vi "DataSocketOutput-Start.vi"(3 "error in (no error)":errorcluster, 4 "OutputRequest\nuser event refnum":T1, 5 "Configuration":T2) -> (0 "error out":errorcluster)   [LabVIEW 2015]
doc: "Starts the DataSocketOutput daemon running.\n\nIf the DataSocket URL is empty, then this will warn the user and then exit."
uses:
  DataSocketOutput-Configuration.ctl
  Typedefs/OutputRequest refnum.ctl
  Typedefs/OutputRequest.ctl
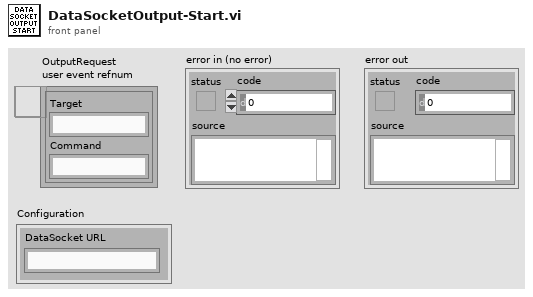
[diagram p1: front panel]
types:
  T1 = typedef "OutputRequest refnum.ctl" = refnum<user-event>
  T2 = typedef "DataSocketOutput-Configuration.ctl" = cluster{"DataSocket URL":string}
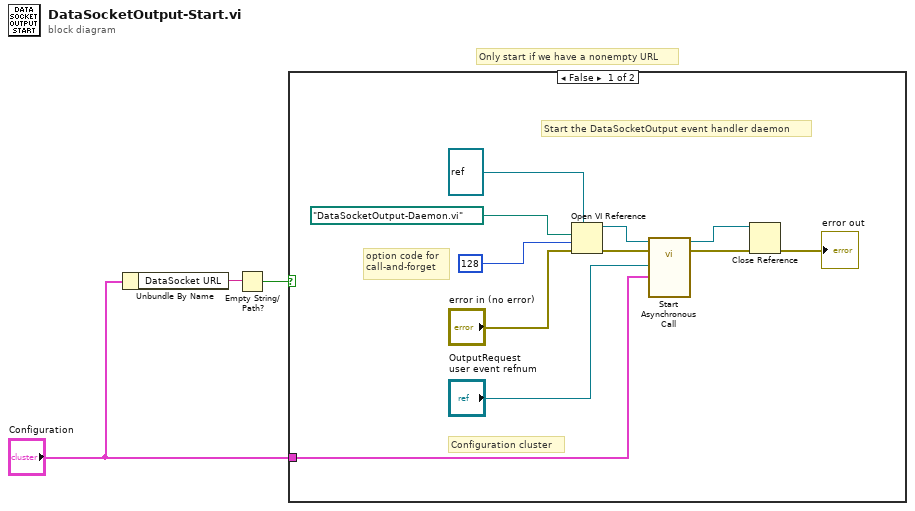
[diagram p0: block diagram]
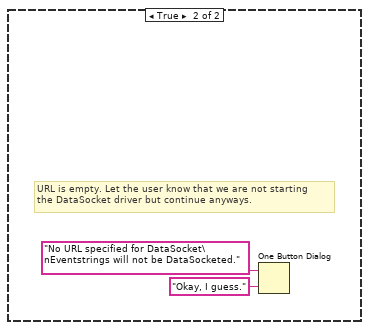
[diagram p2: hidden frame]
diagram:
  # "Only start if we have a nonempty URL"
  n1 = Unbundle By Name("Configuration") -> ("DataSocket URL"=w3:string)
  n2 = Empty String/Path?(string/path=w3) -> (empty?=w2:bool)
  n3 = case shown="False" w2 {
    tunnel: "Configuration" -> [w4 _]
    frame False {
      # "Configuration cluster"
      # "option code for\ncall-and-forget"
      # "Start the DataSocketOutput event handler daemon"
      n4 = Open VI Reference(type specifier VI Refnum (for type only)=refnum<vi> refnum, vi path=path "DataSocketOutput-Daemon.vi", options=128, error in (no error)="error in (no error)") -> (vi reference=w13:refnum<vi>, error out=w14:errorcluster)  [unwired: 2 in]
      n5 = call-by-ref "Start Asynchronous Call"(reference=w13, error in=w14, "Configuration"=w4, "OutputRequest\nuser event refnum"="OutputRequest\nuser event refnum") -> (reference out=w9:refnum<vi>, error out=w10:errorcluster)  [unwired: 3 in]
      n6 = Close Reference(reference=w9, error in (no error)=w10) -> (error out=→"error out":errorcluster)
    }
    frame True {
      # "URL is empty. Let the user know that we are not starting \nthe DataSocket driver but continue anyways."
      n7 = One Button Dialog(message="No URL specified for DataSocket\nEventstrings will not be DataSocketed.", button name ("OK")="Okay, I guess.") -> ()  [unwired: 1 out]
    }
  }
